vi "ValorAuto.vi"(11 "Steps":dbl[][](array[numeric])) -> ()   [LabVIEW 2017]
uses:
  Lift States.ctl
  Cube States.ctl
  Robot Global Data.vi
panel:
  in  "Max Drive Speed":dbl=0.8
  in  "Minimum Drive Speed":dbl=0.15
  out "Step Start Time":u32
  in  "First Time?":bool=TRUE
  in  "Step":i32
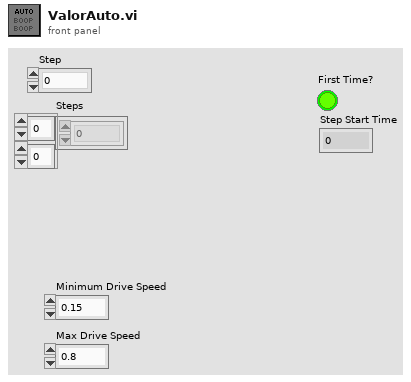
[diagram p1: front panel]
types:
  T1 = typedef "Auto Actions.ctl" = enum16{"Idle", "Drive", "Turn", "Lift", "Cube"}
  T2 = typedef "Lift States.ctl" = enum16{"Manual", "Scale Low", "Scale Middle", "Scale High", "Rock Bottom", "Almost Down"}
  T3 = typedef "Cube States.ctl" = enum16{"Set Motors", "Angle Down", "Angle Up", "Arms In", "Arms Out"}
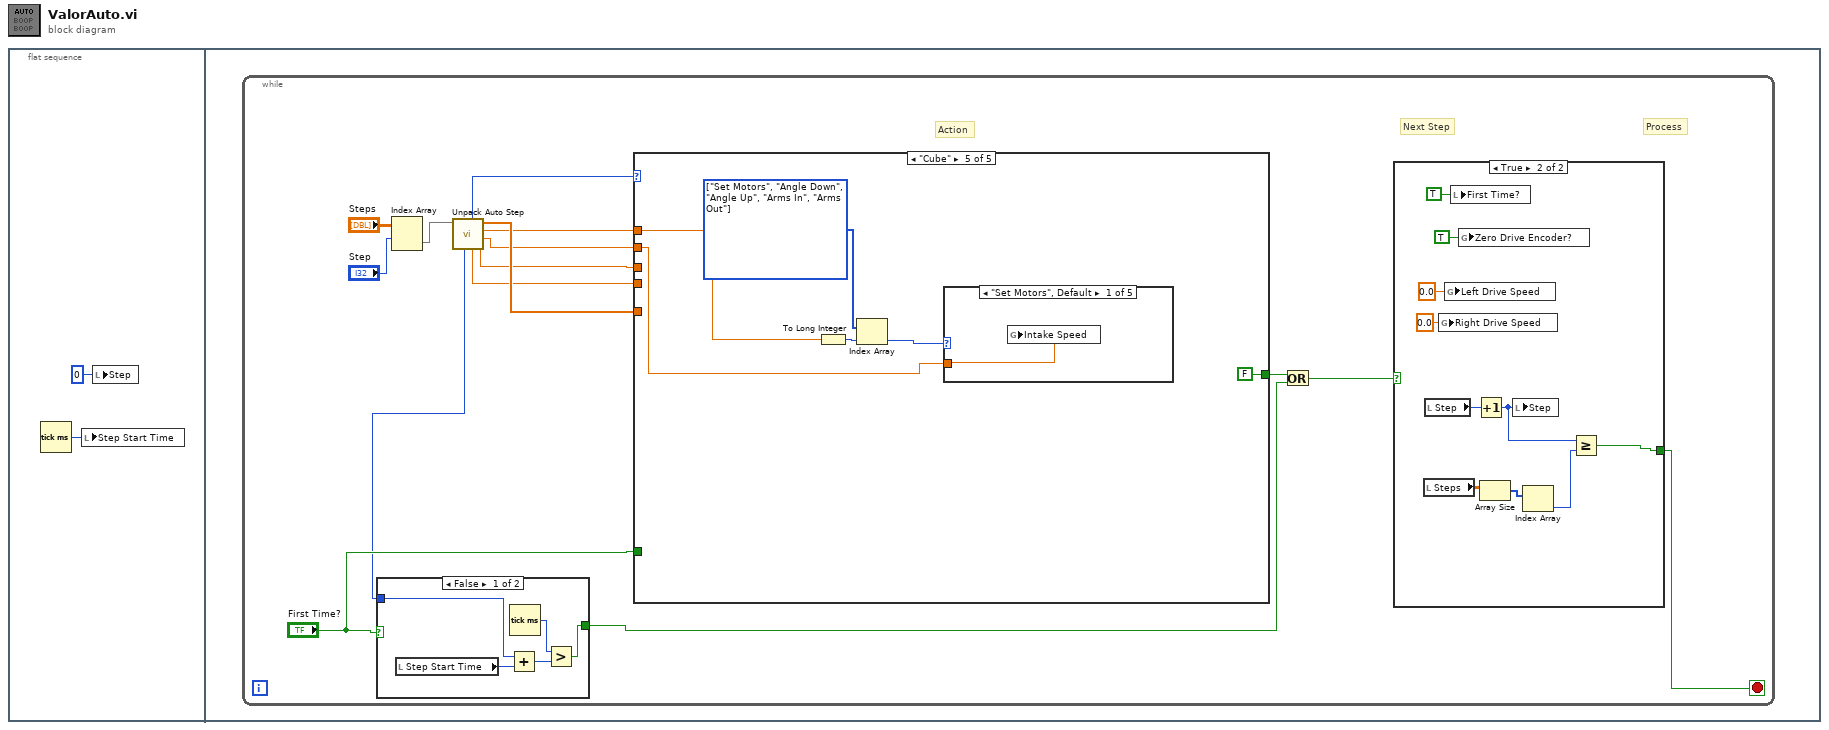
[diagram p0: block diagram]
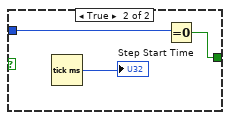
[diagram p2: hidden frame]
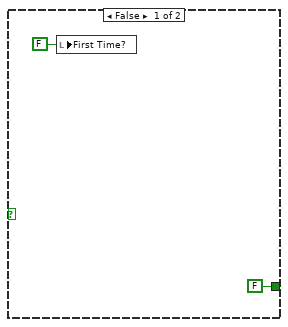
[diagram p3: hidden frame]
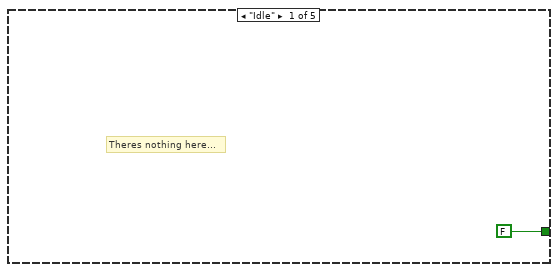
[diagram p4: hidden frame]
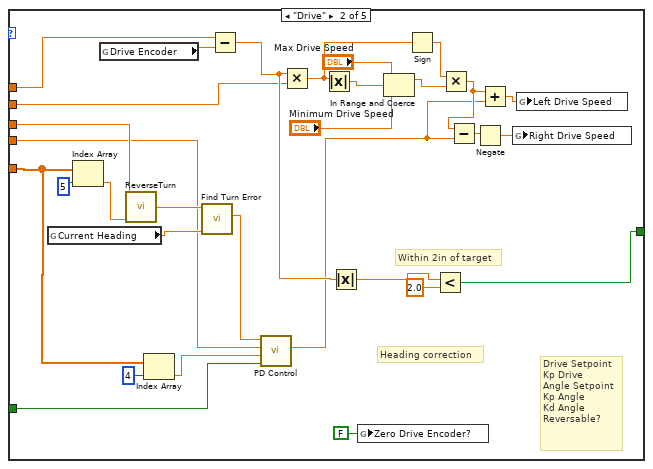
[diagram p5: hidden frame]
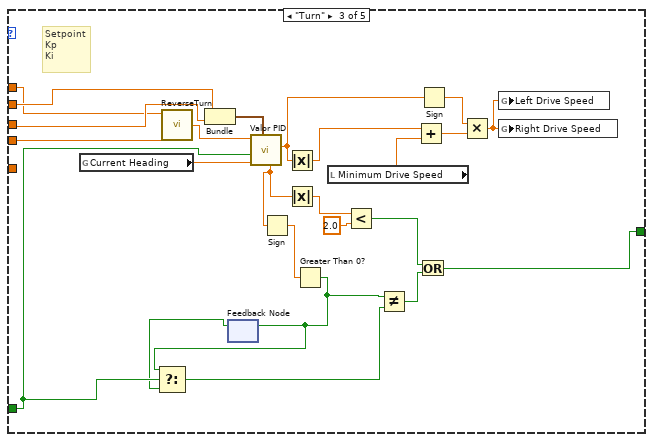
[diagram p6: hidden frame]
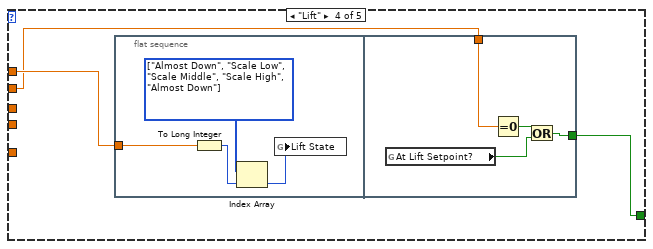
[diagram p7: hidden frame]
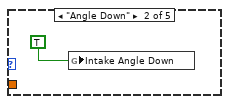
[diagram p8: hidden frame]
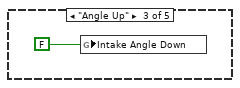
[diagram p9: hidden frame]
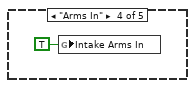
[diagram p10: hidden frame]
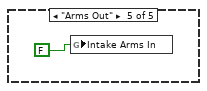
[diagram p11: hidden frame]
diagram:
  n1 = flat-sequence {
    frame #0 {
      n2 = Tick Count (ms)() -> (millisecond timer value=w1:u32)
      n3 = local write "Step Start Time"(w1) -> ()
      n4 = local write "Step"(0 ("Step")) -> ()
    }
    frame #1 {
      n5 = while {
        stop <- w12 stop-if-true
        # "Process"
        # "Next Step"
        # "Action"
        n6 = Index Array(array="Steps", index (row)="Step") -> (element=w10:dbl[])  [unwired: 1 in]
        n7 = call "Unpack Auto Step.vi"("Step Array"=w10) -> ("Arg3"=w6:dbl, "Arg2"=w7:dbl, "Arg1"=w8:dbl, "Args"=w9:dbl[], "Arg4"=w4:dbl, "Step Type"=w3:T1, "Timeout"=w5:u32)  [unwired: 4 in]
        n8 = case shown="False" "First Time?" {
          tunnel: [w19 w24] -> w14
          tunnel: w5 -> [w18 w23]
          frame False {
            n9 = local read "Step Start Time"() -> (w22:u32)
            n10 = Add(x=w18, y=w22) -> (x+y=w21:u32)
            n11 = Tick Count (ms)() -> (millisecond timer value=w20:u32)
            n12 = Greater?(x=w20, y=w21) -> (0:w19:bool)
          }
          frame True {
            n13 = Tick Count (ms)() -> (millisecond timer value=→"Step Start Time":u32)
            n14 = Equal To 0?(x=w23) -> (x = 0?=w24:bool)
          }
        }
        n15 = case shown="\"Cube\"" w3 {
          tunnel: [FALSE w56 w74 w93 FALSE] -> w15
          tunnel: "First Time?" -> [_ w45 w72 _ _]
          tunnel: w9 -> [_ w43 _ _ _]
          tunnel: w8 -> [_ w53 w79 w95 w107]
          tunnel: w7 -> [_ w52 w91 w94 w104]
          tunnel: w6 -> [_ w48 w90 _ _]
          tunnel: w4 -> [_ w39 w80 _ _]
          frame "Idle" {
            # "Theres nothing here..."
          }
          frame "Drive" {
            # "Drive Setpoint\nKp Drive\nAngle Setpoint\nKp Angle\nKd Angle\nReversable?"
            # "Heading correction"
            # "Within 2in of target"
            n16 = global read "Robot Global Data.vi" "Current Heading"() -> (w67:dbl)
            n17 = Index Array(array=w43, index=5) -> (element=w46:dbl)
            n18 = global read "Robot Global Data.vi" "Drive Encoder"() -> (w68:dbl)
            n19 = call "ReverseTurn.vi"("Start Angle"=w48, "Reversable Index"=w46) -> ("Target Angle"=w47:dbl)  [unwired: 6 in]
            n20 = Index Array(array=w43, index=4) -> (element=w41:dbl)
            n21 = call "Find Turn Error.vi"("Target Angle"=w47, "Current Angle"=w67) -> ("Error"=w44:dbl)  [unwired: 7 in]
            n22 = Subtract(x=w53, y=w68) -> (x-y=w55:dbl)
            n23 = call "PD Control.vi"("First Run?"=w45, "kD"=w41, "kP"=w39, "Error"=w44) -> ("PD"=w40:dbl)  [unwired: 7 in]
            n24 = Multiply(x=w55, y=w52) -> (x*y=w63:dbl)
            n25 = Absolute Value(x=w63) -> (abs(x)=w64:dbl)
            n26 = Absolute Value(x=w55) -> (abs(x)=w54:dbl)
            n27 = global write "Robot Global Data.vi" "Zero Drive Encoder?"(FALSE ("Zero Drive Encoder?")) -> ()
            n28 = In Range and Coerce(upper limit="Max Drive Speed", x=w64, lower limit="Minimum Drive Speed") -> (coerced(x)=w62:dbl)  [unwired: 1 out]
            n29 = Sign(1:w63) -> (0:w61:dbl)
            n30 = Less?(x=w54, y=2.0) -> (x < y?=w56:bool)
            n31 = Multiply(x=w61, y=w62) -> (x*y=w58:dbl)
            n32 = Subtract(x=w58, y=w40) -> (x-y=w59:dbl)
            n33 = Negate(x=w59) -> (-x=w66:dbl)
            n34 = Add(x=w58, y=w40) -> (x+y=w60:dbl)
            n35 = global write "Robot Global Data.vi" "Right Drive Speed"(w66) -> ()
            n36 = global write "Robot Global Data.vi" "Left Drive Speed"(w60) -> ()
          }
          frame "Turn" {
            # "Setpoint\nKp\nKi"
            n37 = global read "Robot Global Data.vi" "Current Heading"() -> (w92:dbl)
            n38 = call "ReverseTurn.vi"("Start Angle"=w79, "Reversable Index"=w80) -> ("Target Angle"=w78:dbl)  [unwired: 6 in]
            n39 = Bundle("Arg2"=w91, "Arg3"=w90) -> (w89:cluster{"Arg2":dbl, "Arg3":dbl})  [unwired: 1 in]
            n40 = feedback #1() -> (w71:bool)  [unwired: 1 in]
            n41 = call "Valor PID.vi"("PI"=w89, "Current"=w92, "First Run"=w72, "Target"=w78) -> ("Output"=w84:dbl, "Error"=w77:dbl)  [unwired: 6 in]
            n42 = Sign(1:w77) -> (0:w76:dbl)
            n43 = Absolute Value(x=w84) -> (abs(x)=w83:dbl)
            n44 = Absolute Value(x=w77) -> (abs(x)=w86:dbl)
            n45 = Greater Than 0?(x=w76) -> (x > 0?=w69:bool)
            n46 = Select(t=w69, s=w72, f=w71) -> (s? t:f=w70:bool)
            n47 = feedback-in #1(w69) -> ()
            n48 = local read "Minimum Drive Speed"() -> (w82:dbl)
            n49 = Less?(x=w86, y=2.0) -> (x < y?=w75:bool)
            n50 = Not Equal?(x=w69, y=w70) -> (x != y?=w73:bool)
            n51 = Add(x=w83, y=w82) -> (x+y=w81:dbl)
            n52 = Or(x=w75, y=w73) -> (x .or. y?=w74:bool)
            n53 = Sign(1:w84) -> (0:w88:dbl)
            n54 = Multiply(x=w88, y=w81) -> (x*y=w87:dbl)
            n55 = global write "Robot Global Data.vi" "Left Drive Speed"(w87) -> ()
            n56 = global write "Robot Global Data.vi" "Right Drive Speed"(w87) -> ()
          }
          frame "Lift" {
            n57 = flat-sequence {
              tunnel: w95 -> [w99]
              tunnel: w94 -> [w101]
              tunnel: [w100] -> w93
              frame #0 {
                w97 = T2[] [enum."Almost Down", enum."Scale Low", enum."Scale Middle", enum."Scale High", enum."Almost Down"] items=["Manual", "Scale Low", "Scale Middle", "Scale High", "Rock Bottom", "Almost Down"]
                n58 = To Long Integer(number=w99) -> (32bit integer=w98:i32)
                n59 = Index Array(array=w97, index=w98) -> (element=w96:T2)
                n60 = global write "Robot Global Data.vi" "Lift State"(w96) -> ()
              }
              frame #1 {
                n61 = global read "Robot Global Data.vi" "At Lift Setpoint?"() -> (w102:bool)
                n62 = Equal To 0?(x=w101) -> (x = 0?=w103:bool)
                n63 = Or(x=w103, y=w102) -> (x .or. y?=w100:bool)
              }
            }
          }
          frame "Cube" {
            w106 = T3[] [enum."Set Motors", enum."Angle Down", enum."Angle Up", enum."Arms In", enum."Arms Out"] items=["Set Motors", "Angle Down", "Angle Up", "Arms In", "Arms Out"]
            n64 = To Long Integer(number=w107) -> (32bit integer=w108:i32)
            n65 = Index Array(array=w106, index=w108) -> (element=w105:T3)
            n66 = case shown="\"Set Motors\", Default" w105 {
              tunnel: w104 -> [w110 _ _ _ _]
              frame "Set Motors", Default {
                n67 = global write "Robot Global Data.vi" "Intake Speed"(w110) -> ()
              }
              frame "Angle Down" {
                n68 = global write "Robot Global Data.vi" "Intake Angle Down"(TRUE ("Intake Angle Up")) -> ()
              }
              frame "Angle Up" {
                n69 = global write "Robot Global Data.vi" "Intake Angle Down"(FALSE ("Intake Angle Up")) -> ()
              }
              frame "Arms In" {
                n70 = global write "Robot Global Data.vi" "Intake Arms In"(TRUE ("Intake Arms In")) -> ()
              }
              frame "Arms Out" {
                n71 = global write "Robot Global Data.vi" "Intake Arms In"(FALSE ("Intake Arms In")) -> ()
              }
            }
          }
        }
        n72 = Or(x=w15, y=w14) -> (x .or. y?=w11:bool)
        n73 = case shown="True" w11 {
          tunnel: [FALSE w30] -> w12
          frame False {
            n74 = local write "First Time?"(FALSE ("First Time?")) -> ()
          }
          frame True {
            n75 = local read "Steps"() -> (w34:dbl[][])
            n76 = local read "Step"() -> (w35:i32)
            n77 = global write "Robot Global Data.vi" "Right Drive Speed"(0.0 ("Left Drive Speed")) -> ()
            n78 = global write "Robot Global Data.vi" "Left Drive Speed"(0.0 ("Left Drive Speed")) -> ()
            n79 = local write "First Time?"(TRUE ("First Time?")) -> ()
            n80 = global write "Robot Global Data.vi" "Zero Drive Encoder?"(TRUE ("Zero Drive Encoder?")) -> ()
            n81 = Increment(x=w35) -> (x+1=w29:i32)
            n82 = Array Size(array=w34) -> (size(s)=w33:i32[])
            n83 = local write "Step"(w29) -> ()
            n84 = Index Array(array=w33) -> (element=w28:i32)  [unwired: 1 in]
            n85 = Greater Or Equal?(x=w29, y=w28) -> (x >= y?=w30:bool)
          }
        }
      }
    }
  }
